vi "distance to target.vi"() -> ()   [LabVIEW 2016]
panel:
  in  "distance to target":dbl
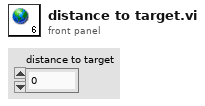
[diagram p1: front panel]
diagram:
